vi "Initiate.vi"(0 "device session in":refnum<class "Device Session.lvclass">, 11 "error in":errorcluster) -> (4 "device session out":refnum<class "Device Session.lvclass">, 15 "error out":errorcluster)   [LabVIEW 2021, in "Device Session.lvclass"]
doc: "Initiates a new acquisition from the FPGA. You must configure the acquisition by running the <B>Configure Acquisition</B> VI before running this VI.\n\n<B>Input Parameters</B>\n\n<B>device session in</B> is a reference to the Device Session object, which contains a session to each instrument design library used in this sample project. This parameter is obtained from the 'Open Session' VI.\n\n<B>error in</B> describes error conditions that occur before this node runs. This input provides standard 'error in' functionality.\n\n<B>Output Parameters</B>\n\n<B>device session out</B> passes a reference to the session to the next VI.\n\n<B>error out</B> contains error information. This output provides standard 'error out' functionality."
uses:
  Device Session.lvclass
  Device Session.lvclass/Device Session.ctl
  <vilib>/Utility/error.llb/Error Cluster From Error Code.vi
  <vilib>/rvi/errors/niLvFpgaAdjustHostInterfaceError.vi
  <vilib>/rvi/interface/nirviReadWriteControl/nirviReadWriteControl.xnode
  FPGA Refnum.ctl
  <instrlib>/_niInstr/Multirecord Acquisition/Interface/v1/Host/niInstr Multirecord Acquisition v1 Host.lvclass
  <instrlib>/HSAI-RIO/Config/Group A/v1/Host/Main/niHSAI Group A Config v1 Host.lvclass
  NiFpgaLv.dll
  <vilib>/rvi/interface/Simulation/niFpgaSimulationCallBeginRW.vi
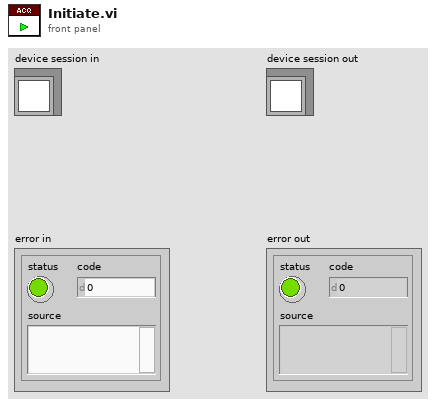
[diagram p1: front panel]
types:
  T1 = typedef "Device Session.lvclass/Device Session Object.ctl" = cluster{"fpga reference":T2, "reg bus":refnum<class "niInstr FIFO Register Bus v1 Host.lvclass">, "subsystem map":refnum<class "niInstr Subsystem Map v1 Host.lvclass">, "cal data":refnum<class "niHSAI Cal Data v1 Host.lvclass">, "config":refnum<class "niHSAI Group A Config v1 Host.lvclass">, "acquisition 0":refnum<class "niInstr Multirecord Acquisition v1 Host.lvclass">, "acquisition 1":refnum<class "niInstr Multirecord Acquisition v1 Host.lvclass">, "number of selected acq channels":u8, "selected acq channels":bool[], "number of channels":u32, "configured channels":bool[], "acq configuration":cluster{"number of samples":u64, "number of records":u64, "pretrigger samples":u64}, "actual channel configuration":T3[], "sample clock rate (Hz)":dbl, "scaling coefficients":T7[]}
  T2 = typedef "Device Session.lvclass/FPGA Refnum.ctl" = refnum<k20>
  T3 = typedef "niHSAI Types v1 Host.lvlib/Channel Configuration.ctl" = cluster{"channel":u32, "coupling":T4, "impedance":T5, "bandwidth":T6, "vertical range":dbl, "vertical offset":dbl}
  T4 = typedef "niHSAI Types v1 Host.lvlib/Coupling.ctl" = enum8{"Default", "DC", "AC"}
  T5 = typedef "niHSAI Types v1 Host.lvlib/Impedance.ctl" = enum8{"Default", "1 mega ohm", "50 ohm"}
  T6 = typedef "niHSAI Types v1 Host.lvlib/Bandwidth.ctl" = enum8{"Default", "Full Bandwidth", "Anti-alias Filter", "150 MHz"}
  T7 = typedef "niInstr Multirecord Acquisition v1 Host.lvclass/Scaling Coefficient.ctl" = cluster{"gain":dbl, "offset":dbl}
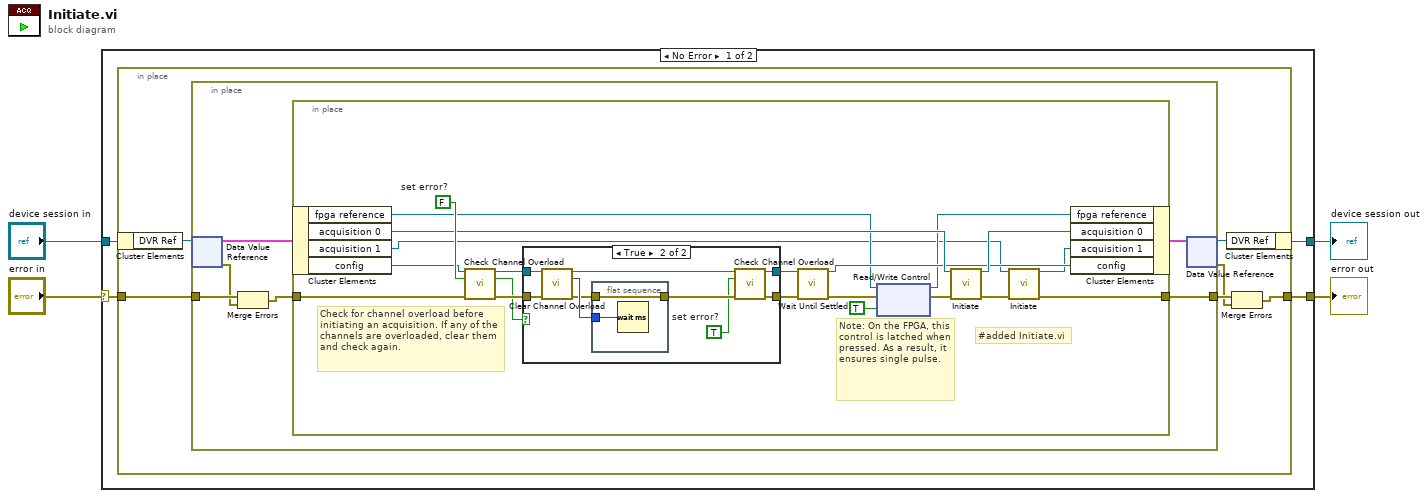
[diagram p0: block diagram]
diagram:
  n1 = case shown="No Error" "error in" {
    selector: "error in" -> [w8 w55]
    tunnel: "device session in" -> [w6 w54]
    tunnel: [w7 w55] -> w2
    tunnel: [w5 w54] -> w1
    frame No Error {
      n2 = in-place {
        in-place-border: w8 -> [w14]
        in-place-border: [w12] -> w7
        n3 = in-place-cluster #1(w6) -> ("DVR Ref"=w10:refnum<data-value>)
        n4 = in-place {
          in-place-border: w14 -> [w19]
          in-place-border: [w20] -> w13
          n5 = in-place-dvr #2(w10) -> (w16:T1, w18:errorcluster)
          n6 = Merge Errors(w19, w18) -> (w17:errorcluster)
          n7 = in-place {
            in-place-border: [w21] -> w20
            in-place-border: w17 -> [w32]
            w40 = FALSE  # set error?
            # "#added Initiate.vi"
            # "Note: On the FPGA, this control is latched when pressed. As a result, it ensures single pulse."
            # "Check for channel overload before initiating an acquisition. If any of the channels are overloaded, clear them and check again."
            n8 = in-place-cluster #3(w16) -> ("fpga reference"=w27:T2, "acquisition 0"=w31:refnum<class "niInstr Multirecord Acquisition v1 Host.lvclass">, "acquisition 1"=w24:refnum<class "niInstr Multirecord Acquisition v1 Host.lvclass">, "config"=w29:refnum<class "niHSAI Group A Config v1 Host.lvclass">)
            n9 = call-dynamic "Check Channel Overload.vi"("session in"=w29, "set error? (T)"=w40, "error in"=w32) -> ("session out"=w39:refnum<class "niHSAI Group A Config v1 Host.lvclass">, "overloaded?"=w25:bool, "error out"=w38:errorcluster)  [unwired: 10 in]
            n10 = case shown="True" w25 {
              tunnel: w39 -> [w42 w51]
              tunnel: [w42 w49] -> w36
              tunnel: w38 -> [w41 w50]
              tunnel: [w41 w48] -> w37
              frame False {
              }
              frame True {
                w43 = TRUE  # set error?
                n11 = call-dynamic "Clear Channel Overload.vi"("session in"=w51, "error in"=w50) -> ("session out"=w44:refnum<class "niHSAI Group A Config v1 Host.lvclass">, "min wait time (ms)"=w47:u32, "error out"=w46:errorcluster)  [unwired: 11 in]
                n12 = flat-sequence {
                  tunnel: w47 -> [w53]
                  tunnel: w46 -> [w52]
                  tunnel: [w52] -> w45
                  frame #0 {
                    n13 = Wait (ms)(milliseconds to wait=w53) -> ()  [unwired: 1 out]
                  }
                }
                n14 = call-dynamic "Check Channel Overload.vi"("session in"=w44, "set error? (T)"=w43, "error in"=w45) -> ("session out"=w49:refnum<class "niHSAI Group A Config v1 Host.lvclass">, "error out"=w48:errorcluster)  [unwired: 10 in, 1 out]
              }
            }
            n15 = call-dynamic "Wait Until Settled.vi"("session in"=w36, "error in"=w37) -> ("session out"=w28:refnum<class "niHSAI Group A Config v1 Host.lvclass">, "error out"=w35:errorcluster)  [unwired: 12 in]
            n16 = xnode "Read/Write Control"("FPGA VI Reference In"=w27, "error in"=w35, "reset"=TRUE) -> ("FPGA VI Reference Out"=w26:T2, "error out"=w34:errorcluster)
            n17 = call-dynamic "Initiate.vi"("session in"=w31, "error in"=w34) -> ("session out"=w30:refnum<class "niInstr Multirecord Acquisition v1 Host.lvclass">, "error out"=w22:errorcluster)  [unwired: 12 in]
            n18 = call-dynamic "Initiate.vi"("session in"=w24, "error in"=w22) -> ("session out"=w23:refnum<class "niInstr Multirecord Acquisition v1 Host.lvclass">, "error out"=w21:errorcluster)  [unwired: 12 in]
            n19 = in-place-cluster #3("fpga reference"=w26, "acquisition 0"=w30, "acquisition 1"=w23, "config"=w28) -> (w15:T1)
          }
          n20 = in-place-dvr #2(w15) -> (w9:refnum<data-value>, w11:errorcluster)
        }
        n21 = in-place-cluster #1("DVR Ref"=w9) -> (w5:refnum<class "Device Session.lvclass">)
        n22 = Merge Errors(w13, w11) -> (w12:errorcluster)
      }
    }
    frame Error {
    }
  }
  "error out" <- w2
  "device session out" <- w1
